vi "setLoadImpedance.vi"(8 "error in (no error)":errorcluster, 10 "Load Impedance":T1=10000000.0 items=["50 Ohm"=50.0, "High Z"=10000000.0], 11 "FgenNiPxi in":refnum<class "ArbNi.lvclass">) -> (0 "error out":errorcluster, 3 "FgenNiPxi out":refnum<class "ArbNi.lvclass">)   [LabVIEW 2023, in "ArbNi.lvclass"]
uses:
  ArbNi.lvclass
  Data/arbLoadImpedance.ctl
  ArbNi.lvclass/ArbNi.ctl
  Arb.lvclass
  sweArb.lvlib
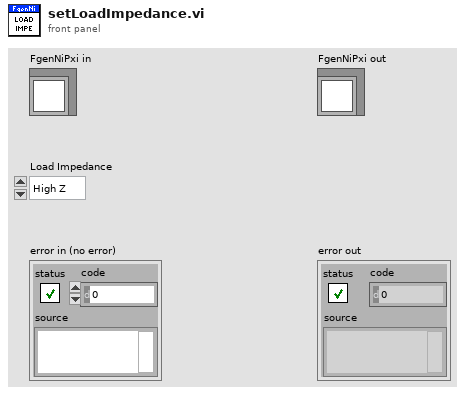
[diagram p1: front panel]
types:
  T1 = typedef "sweArb.lvlib/arbLoadImpedance.ctl" = dbl
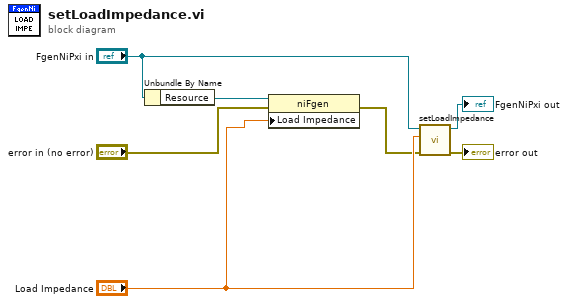
[diagram p0: block diagram]
diagram:
  n1 = Unbundle By Name("FgenNiPxi in") -> ("Resource"=w3:refnum<k15>)
  n2 = property class="niFgen"(reference=w3, error in="error in (no error)", "Load Impedance"="Load Impedance") -> (error out=w1:errorcluster)  [unwired: 1 out]
  n3 = call-parent "setLoadImpedance.vi"("error in (no error)"=w1, "Load Impedance"="Load Impedance", "Fgen in"="FgenNiPxi in") -> ("error out"=→"error out":errorcluster, "Fgen out"=→"FgenNiPxi out":refnum<class "ArbNi.lvclass">)  [unwired: 7 in]
